vi "Clear Framebuffer.vi"(11 "Data Value Reference in":refnum<data-value>) -> (3 "Data Value Reference out":refnum<data-value>)   [LabVIEW 2020, in "3D.lvlib"]
uses:
  3D.lvlib
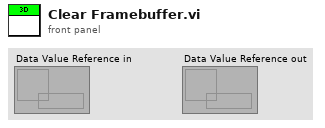
[diagram p1: front panel]
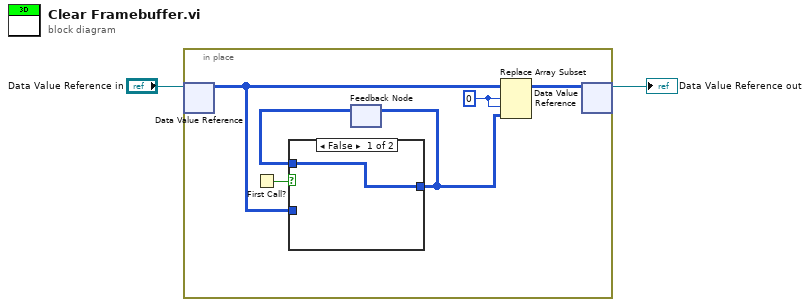
[diagram p0: block diagram]
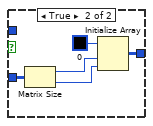
[diagram p2: hidden frame]
diagram:
  n1 = in-place {
    w6 = 0 ("index (row)")
    n2 = in-place-dvr #1("Data Value Reference in") -> (w7:u32[][])  [unwired: 1 out]
    n3 = First Call?() -> (First Call?: T/F=w5:bool)
    n4 = feedback #2() -> (w3:u32[][])  [unwired: 1 in]
    n5 = case shown="False" w5 {
      tunnel: w7 -> [_ w14]
      tunnel: [w9 w12] -> w4
      tunnel: w3 -> [w9 _]
      frame False {
      }
      frame True {
        n6 = Matrix Size(0:w14) -> (1:w11:i32, 2:w10:i32)
        n7 = Initialize Array(u32 0 ("Fill Colour"), w11, w10) -> (w12:u32[][])
      }
    }
    n8 = feedback-in #2(w4) -> ()
    n9 = Replace Array Subset(array=w7, new element=w4, index (row)=w6, index (col)=w6) -> (w8:u32[][])
    n10 = in-place-dvr #1(w8) -> (→"Data Value Reference out":refnum<data-value>)  [unwired: 1 out]
  }
